vi "create_data_to_send.vi"(8 "error in (no error)":errorcluster, 9 "data":u8, 10 "address":u8, 11 "command":u8) -> (0 "error out":errorcluster, 1 "send byte":u8[](array[numeric]), 2 "send string":string, 4 "crc":u8)   [LabVIEW 2018]
doc: "creates a string and a byte array from the command, board and data settings. CRC is calculated internally"
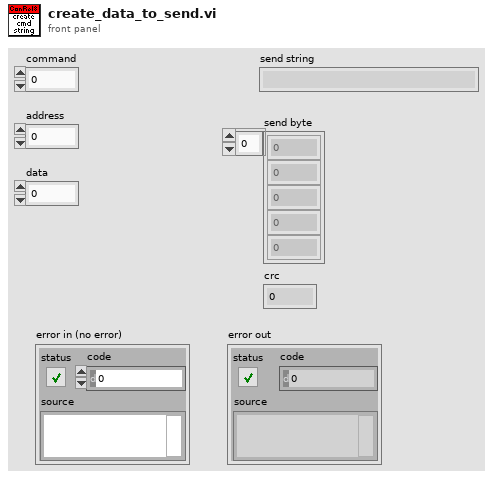
[diagram p1: front panel]
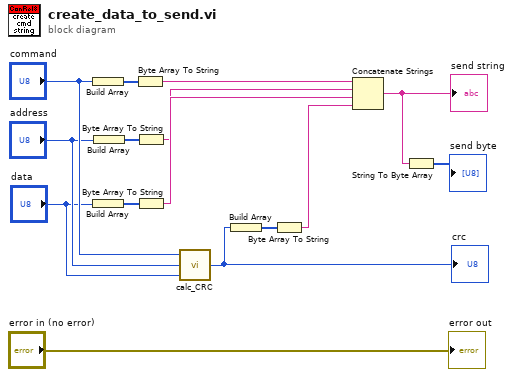
[diagram p0: block diagram]
diagram:
  n1 = Build Array("command") -> (w7:u8[])
  n2 = Build Array("data") -> (w5:u8[])
  n3 = Build Array("address") -> (w6:u8[])
  n4 = Byte Array To String(unsigned byte array=w7) -> (string=w10:string)
  n5 = Byte Array To String(unsigned byte array=w6) -> (string=w11:string)
  n6 = Byte Array To String(unsigned byte array=w5) -> (string=w12:string)
  n7 = call "calc_CRC.vi"("data"="data", "address"="address", "command"="command") -> ("CRC"=w9:u8)
  "crc" <- w9
  n8 = Build Array(w9) -> (w8:u8[])
  n9 = Byte Array To String(unsigned byte array=w8) -> (string=w13:string)
  n10 = Concatenate Strings(w10, w11, w12, w13) -> (w14:string)
  "send string" <- w14
  n11 = String To Byte Array(string=w14) -> (unsigned byte array=→"send byte":u8[])
  "error out" <- "error in (no error)"
